vi "ImpactCheck.vi"(11 "Numeric":i32) -> (0 "Start":u32, 1 "Impact":u32, 2 "Thermal":u32, 3 "Gas Detected":u32)   [LabVIEW 2020]
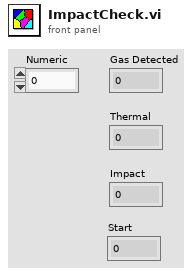
[diagram p1: front panel]
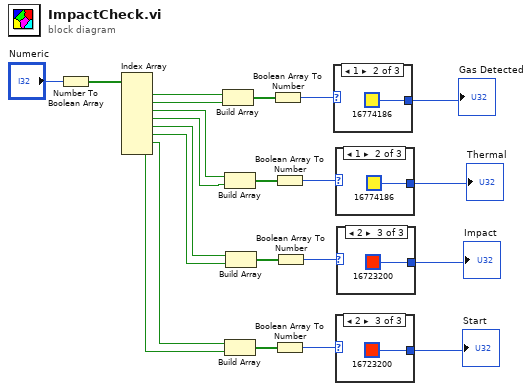
[diagram p0: block diagram]
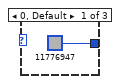
[diagram p2: hidden frame]
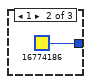
[diagram p3: hidden frame]
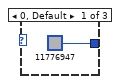
[diagram p4: hidden frame]
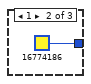
[diagram p5: hidden frame]
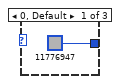
[diagram p6: hidden frame]
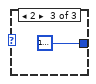
[diagram p7: hidden frame]
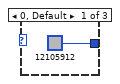
[diagram p8: hidden frame]
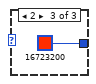
[diagram p9: hidden frame]
diagram:
  n1 = Number To Boolean Array(number="Numeric") -> (Boolean array=w10:bool[])
  n2 = Index Array(array=w10) -> (element #1=w9:bool, element #2=w8:bool, element #3=w17:bool, element #4=w18:bool, element #5=w19:bool, element #6=w20:bool, element #7=w2:bool, element #8=w1:bool)  [unwired: 8 in]
  n3 = Build Array(w9, w8) -> (w7:bool[])
  n4 = Build Array(w17, w18) -> (w14:bool[])
  n5 = Build Array(w2, w1) -> (w4:bool[])
  n6 = Build Array(w19, w20) -> (w16:bool[])
  n7 = Boolean Array To Number(Boolean array=w7) -> (number=w6:u32)
  n8 = Boolean Array To Number(Boolean array=w14) -> (number=w13:u32)
  n9 = Boolean Array To Number(Boolean array=w4) -> (number=w3:u32)
  n10 = Boolean Array To Number(Boolean array=w16) -> (number=w15:u32)
  n11 = case shown="1" w6 {
    tunnel: [u32 12105912 ("Gas Detected") u32 16774186 ("Gas Detected") u32 16723200 ("Gas Detected")] -> w12
    frame 0, Default {
    }
    frame 1 {
    }
    frame 2 {
    }
  }
  "Gas Detected" <- w12
  n12 = case shown="1" w13 {
    tunnel: [u32 11776947 ("Gas Detected") u32 16774186 ("Gas Detected") u32 16777224 ("Gas Detected")] -> w21
    frame 0, Default {
    }
    frame 1 {
    }
    frame 2 {
    }
  }
  "Thermal" <- w21
  n13 = case shown="2" w3 {
    tunnel: [u32 11776947 ("Gas Detected") u32 16774186 ("Gas Detected") u32 16723200 ("Gas Detected")] -> w5
    frame 0, Default {
    }
    frame 1 {
    }
    frame 2 {
    }
  }
  "Start" <- w5
  n14 = case shown="2" w15 {
    tunnel: [u32 11776947 ("Gas Detected") u32 16774186 ("Gas Detected") u32 16723200 ("Gas Detected")] -> w22
    frame 0, Default {
    }
    frame 1 {
    }
    frame 2 {
    }
  }
  "Impact" <- w22
